vi "IO_Export_Spectra_To_Spreadsheet.vi"(4 "header? (write header:T)":bool=TRUE, 5 "delimiter (Tab)":string="\t", 7 "operation (0:open)":T1(ring)=enum."replace or create", 9 "multiple time columns? (single:F)":bool, 10 "Array 2":cluster{"f0":dbl, "df":dbl, "magnitude":dbl[]}[](array[cluster]), 11 "file path (dialog if empty)":path) -> ()   [LabVIEW 2011]
doc: "Converts a waveform to a text string and writes the string to a new byte stream file or appends the string to an existing file. Wire data to the <B>Waveform</B> input to determine the polymorphic instance to use or manually select the instance."
panel:
  out "spreadsheet string":string
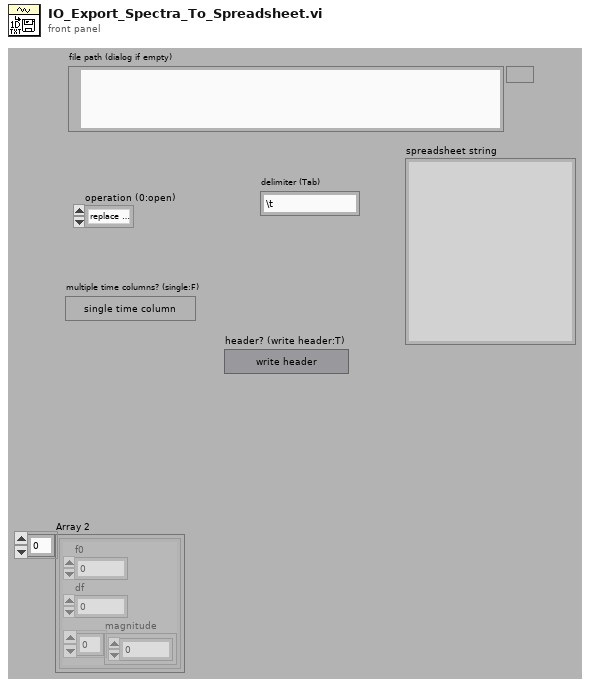
[diagram p1: front panel]
types:
  T1 = enum16{"open", "replace", "create", "open or create", "replace or create", "replace or create with confirmation"}
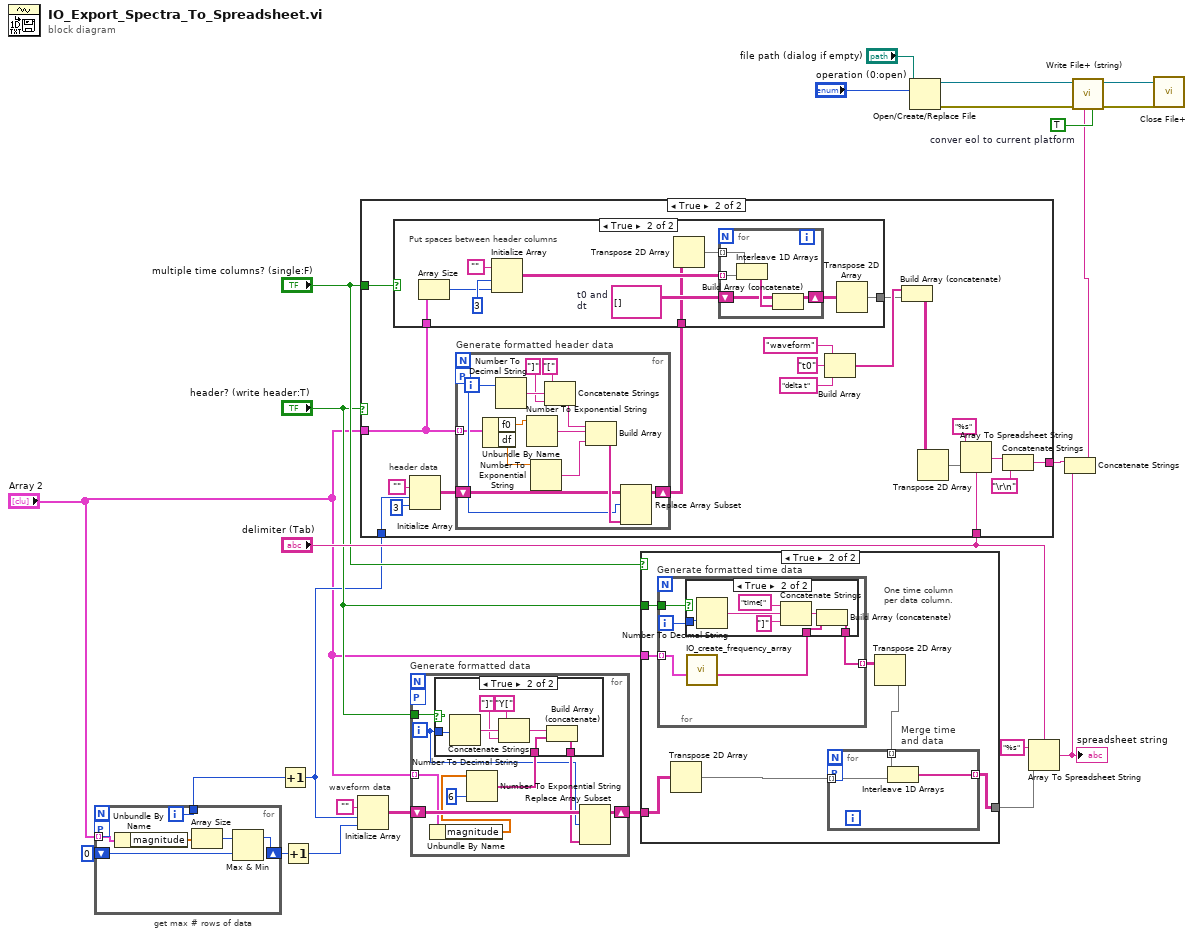
[diagram p0: block diagram]
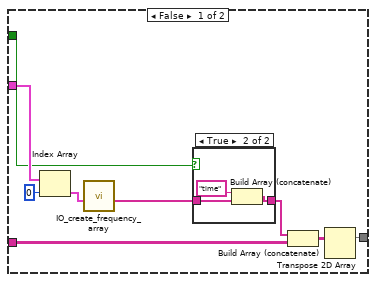
[diagram p2: hidden frame]
diagram:
  w21 = TRUE  # conver eol to current platform
  # "waveform data"
  # "get max # rows of data"
  n1 = for {
    tunnel: "Array 2" -> [w26] mode=indexing
    shift-right: [w28] -> w7
    shift-left: 0 -> [w29]
    tunnel: [w27] -> w5
    workers-P: _ -> [_]
    i -> [w27]
    n2 = Unbundle By Name(w26) -> ("magnitude"=w25:dbl[])
    n3 = Array Size(array=w25) -> (size(s)=w30:i32)
    n4 = Max & Min(x=w30, y=w29) -> (max(x,y)=w28:i32)  [unwired: 1 out]
  }
  n5 = Increment(x=w5) -> (x+1=w4:i32)
  n6 = Increment(x=w7) -> (x+1=w3:i32)
  n7 = Initialize Array("", w4, w3) -> (w6:string[][])
  n8 = case shown="True" "header? (write header:T)" {
    tunnel: "delimiter (Tab)" -> [_ w47]
    tunnel: "Array 2" -> [_ w41]
    tunnel: [_ w42] -> w14
    tunnel: "multiple time columns? (single:F)" -> [_ w39]
    tunnel: w4 -> [_ w32]
    frame False {
    }
    frame True {
      # "header data"
      n9 = Initialize Array("", w32, 3 ("dimension size")) -> (w31:string[][])
      n10 = for "Generate formatted header data" {
        tunnel: w41 -> [w70] mode=indexing
        shift-right: [w72] -> w37
        shift-left: w31 -> [w73]
        workers-P: _ -> [_]
        i -> [w71]
        n11 = Unbundle By Name(w70) -> ("f0"=w69:dbl, "df"=w67:dbl)
        n12 = Number To Decimal String(number=w71) -> (decimal integer string=w77:string)  [unwired: 1 in]
        n13 = Number To Exponential String(number=w69) -> (E-format string=w68:string)  [unwired: 3 in]
        n14 = Number To Exponential String(number=w67) -> (E-format string=w66:string)  [unwired: 3 in]
        n15 = Concatenate Strings("[", w77, "]") -> (w78:string)
        n16 = Build Array(w78, w68, w66) -> (w74:string[])
        n17 = Replace Array Subset(array=w73, new element=w74, index (row)=w71) -> (w72:string[][])  [unwired: 1 in]
      }
      n18 = case shown="True" w39 {
        tunnel: w41 -> [_ w60]
        tunnel: [w50 w55] -> w38
        tunnel: w37 -> [w50 w54]
        frame False {
          # "Leave the header data alone"
        }
        frame True {
          w58 = string[][] []  # t0 and dt
          # "Put spaces between header columns"
          n19 = Array Size(array=w60) -> (size(s)=w51:i32)
          n20 = Initialize Array("", 3 ("Dimension Size"), w51) -> (w57:string[][])
          n21 = Transpose 2D Array(2D array=w54) -> (transposed array=w53:string[][])
          n22 = for {
            shift-right: [w62] -> w56
            shift-left: w58 -> [w63]
            tunnel: w57 -> [w65] mode=indexing
            tunnel: w53 -> [w61] mode=indexing
            n23 = Interleave 1D Arrays(w61, w65) -> (w64:string[])
            n24 = Build Array (concatenate)(w63, w64) -> (w62:string[][])
          }
          n25 = Transpose 2D Array(2D array=w56) -> (transposed array=w55:string[][])
        }
      }
      n26 = Build Array("waveform", "t0", "delta t") -> (w40:string[])
      n27 = Build Array (concatenate)(w40, w38) -> (w35:string[][])
      n28 = Transpose 2D Array(2D array=w35) -> (transposed array=w36:string[][])
      n29 = Array To Spreadsheet String(delimiter (Tab)=w47, array=w36, 3:"%s" ("format string")) -> (spreadsheet string=w44:string)
      n30 = Concatenate Strings(w44, "\r\n") -> (w42:string)
    }
  }
  n31 = for "Generate formatted data" {
    tunnel: "Array 2" -> [w80] mode=indexing
    tunnel: "header? (write header:T)" -> [w84]
    shift-right: [w85] -> w13
    shift-left: w6 -> [w86]
    workers-P: _ -> [_]
    i -> [w81]
    n32 = Unbundle By Name(w80) -> ("magnitude"=w79:dbl[])
    n33 = Number To Exponential String(number=w79, precision (6)=i16 6) -> (E-format string=w83:string[])  [unwired: 2 in]
    n34 = case shown="True" w84 {
      tunnel: w81 -> [_ w92]
      tunnel: w83 -> [w88 w90]
      tunnel: [w88 w89] -> w82
      frame False {
      }
      frame True {
        n35 = Number To Decimal String(number=w92) -> (decimal integer string=w95:string)  [unwired: 1 in]
        n36 = Concatenate Strings("Y[", w95, "]") -> (w91:string)
        n37 = Build Array (concatenate)(w91, w90) -> (w89:string[])
      }
    }
    n38 = Replace Array Subset(array=w86, new element=w82, index (row)=w81) -> (w85:string[][])  [unwired: 1 in]
  }
  n39 = case shown="True" "multiple time columns? (single:F)" {
    tunnel: "Array 2" -> [w100 w115]
    tunnel: w13 -> [w103 w113]
    tunnel: [w101 w109] -> w12
    tunnel: "header? (write header:T)" -> [w98 w110]
    frame False {
      # "One time column - check for equal dt and t0"
      n40 = Index Array(array=w100, index=0 ("Index")) -> (element=w97:cluster{"f0":dbl, "df":dbl, "magnitude":dbl[]})
      n41 = call "IO_create_frequency_array.vi"("cor"=w97) -> ("Array 2"=w96:string[])  [unwired: 10 in]
      n42 = case shown="True" w98 {
        tunnel: w96 -> [w105 w108]
        tunnel: [w105 w107] -> w99
        frame False {
        }
        frame True {
          n43 = Build Array (concatenate)("time", w108) -> (w107:string[])
        }
      }
      n44 = Build Array (concatenate)(w99, w103) -> (w102:string[][])
      n45 = Transpose 2D Array(2D array=w102) -> (transposed array=w101:string[][])
    }
    frame True {
      # "One time column\nper data column."
      n46 = for "Generate formatted time data" {
        tunnel: [w121] -> w114 mode=indexing
        tunnel: w115 -> [w120] mode=indexing
        tunnel: w110 -> [w122]
        i -> [w123]
        n47 = call "IO_create_frequency_array.vi"("cor"=w120) -> ("Array 2"=w119:string[])  [unwired: 10 in]
        n48 = case shown="True" w122 {
          tunnel: w123 -> [_ w128]
          tunnel: w119 -> [w124 w126]
          tunnel: [w124 w125] -> w121
          frame False {
          }
          frame True {
            n49 = Number To Decimal String(number=w128) -> (decimal integer string=w131:string)  [unwired: 1 in]
            n50 = Concatenate Strings("time[", w131, "]") -> (w127:string)
            n51 = Build Array (concatenate)(w127, w126) -> (w125:string[])
          }
        }
      }
      n52 = Transpose 2D Array(2D array=w113) -> (transposed array=w112:string[][])
      n53 = Transpose 2D Array(2D array=w114) -> (transposed array=w111:string[][])
      n54 = for "Merge time\nand data" {
        tunnel: w112 -> [w118] mode=indexing
        tunnel: w111 -> [w117] mode=indexing
        tunnel: [w116] -> w109 mode=indexing
        workers-P: _ -> [_]
        n55 = Interleave 1D Arrays(w117, w118) -> (w116:string[])
      }
    }
  }
  n56 = Open/Create/Replace File(file path (use dialog)="file path (dialog if empty)", operation (0:open)="operation (0:open)") -> (refnum out=w17:refnum<file>, error out=w18:errorcluster)  [unwired: 4 in, 1 out]
  n57 = Array To Spreadsheet String(delimiter (Tab)="delimiter (Tab)", array=w12, 3:"%s" ("format (%.3f)")) -> (spreadsheet string=w16:string)
  "spreadsheet string" <- w16
  n58 = Concatenate Strings(w14, w16) -> (w15:string)
  n59 = call <vilib>:"Write File+ (string).vi"("convert eol? (no:F)"=w21, "string"=w15, "error in (no error)"=w18, "refnum"=w17) -> ("error out"=w24:errorcluster, "dup refnum"=w22:refnum<file>)  [unwired: 3 in, 1 out]
  n60 = call <vilib>:"Close File+.vi"("error in (no error)"=w24, "refnum"=w22) -> ()  [unwired: 3 in, 3 out]
